vi "ToString_ReturnsVITitle.vi"() -> ()   [LabVIEW 2019, in "TestCaseTest.lvlib" / "Fact.lvlib"]
uses:
  Fact.lvlib
  a7e9dbe7-fcdc-4991-af27-9af2d0a95db2.vi
  TestCase/Fact/Fact.lvclass
  Constraint/IsEqual/IsEqual.lvclass
  TestCaseTestSupport/TestCaseTestSupport.lvlib
panel:
  out "error out":errorcluster
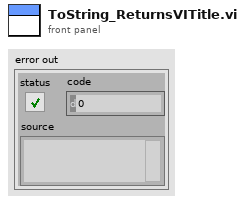
[diagram p1: front panel]
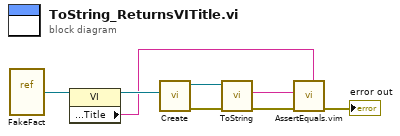
[diagram p0: block diagram]
diagram:
  n1 = vi-ref "FakeFact.vi"() -> (w4:refnum<vi>)
  n2 = property class="VI"(reference=w4) -> (reference out=w3:refnum<vi>, "Front Panel.Title"=w1:string)  [unwired: 1 in, 1 out]
  n3 = call "Create.vi"("VI Refnum"=w3) -> ("error out"=w7:errorcluster, "Fact"=w8:refnum<class "Fact.lvclass">)  [unwired: 9 in]
  n4 = call-dynamic "ToString.vi"("error in (no error)"=w7, "Fact in"=w8) -> ("error out"=w6:errorcluster, "String"=w2:string)  [unwired: 7 in, 1 out]
  n5 = call "AssertEquals.vim"("Expected"=w1, "error in (no error)"=w6, "Actual"=w2) -> ("error out"=→"error out":errorcluster)  [unwired: 8 in]
